vi "PV ModulLine config relay.vi"(8 "error in (no error)":errorcluster, 9 "PV ModulLine config relay - Cluster":T1={"Parameter"=enum." Configuration Relais 1 (045)", "Parameter\nread only<->describe"=FALSE, "Configuration R1 .. R6"=9, "Pressure switch point (hPa)"=1.0000000005} {"Pressure switch point (hPa)" min=5e-10 max=2000.0 step=1.0 format="%_3e"; "Configuration R1 .. R6" items=["0 = rot. speed switch point attained", "1 = no error", "2 = error", "3 = warning", "4 = error and/or warning", "5 = set speed attained", "6 = pump on", "7 = pump accelerates", "8 = pump decelerater", "9 = always 0 (off)", "10 = always 1 (on)", "11 = remote priority active", "12 = heating", "13 = backing pump", "14 = sealing gas", "15 = pumping station", "16 = pump rotates", "17 = pump does not rotate", "18 = TMS temperature engaged  ", "19 = Pressure below pressure switchpoint 1", "20 = Pressure below pressure switchpoint 2", "21 = Pressure below pressure switchpoint 3", "22 = Pressure below pressure switchpoint 4"]}, 10 "Adress of unit":u16=10 max=999 step=1, 11 "VISA session":refnum<visa-resource-name>) -> (0 "error out":errorcluster, 2 "response (data)":string, 3 "dup VISA session":refnum<visa-resource-name>)   [LabVIEW 2021, in "Pfeiffer Vacuum.lvlib"]
doc: "There are 6 parameters available, only one of which can be enabled at a time. \n\n Configuration Relais 1 (045)\n Configuration Relais 2 (046)\n Configuration Relais 3 (047)\n Configuration Relais 4 (048)\n Pressure switch point 1 [mbar] (730)\n Pressure switch point 2 [mbar] (732) \n\n \nNote: Any settings for an parameter that is not selected will be ignored. If a value is out of range, it will be changed to either the upper or the lower limit of the range."
uses:
  <instrlib>/Pfeiffer Vacuum/Pfeiffer Vacuum.lvlib
  <instrlib>/Pfeiffer Vacuum/Public/ModulLine/PV ModulLine config relay - Cluster.ctl
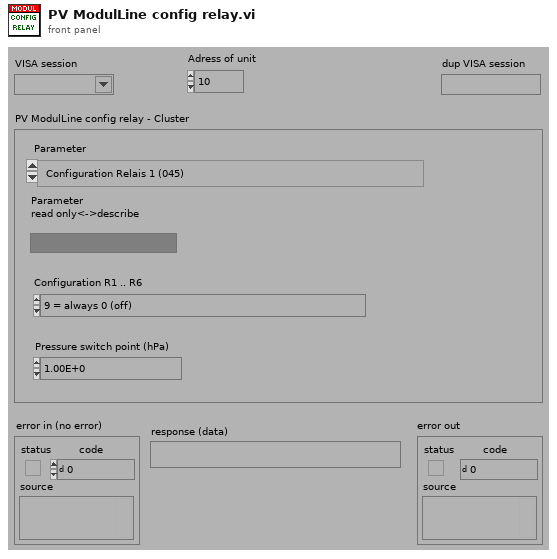
[diagram p1: front panel]
types:
  T1 = typedef "Pfeiffer Vacuum.lvlib/PV ModulLine config relay - Cluster.ctl" = cluster{"Parameter":enum16{" Configuration Relais 1 (045)", " Configuration Relais 2 (046)", " Configuration Relais 3 (047)", " Configuration Relais 4 (048)", " Pressure switch point 1 [mbar] (730)", " Pressure switch point 2 [mbar] (732)"}, "Parameter\nread only<->describe":bool, "Configuration R1 .. R6":u16, "Pressure switch point (hPa)":dbl}
  T2 = enum16{" Configuration Relais 1 (045)", " Configuration Relais 2 (046)", " Configuration Relais 3 (047)", " Configuration Relais 4 (048)", " Pressure switch point 1 [mbar] (730)", " Pressure switch point 2 [mbar] (732)"}
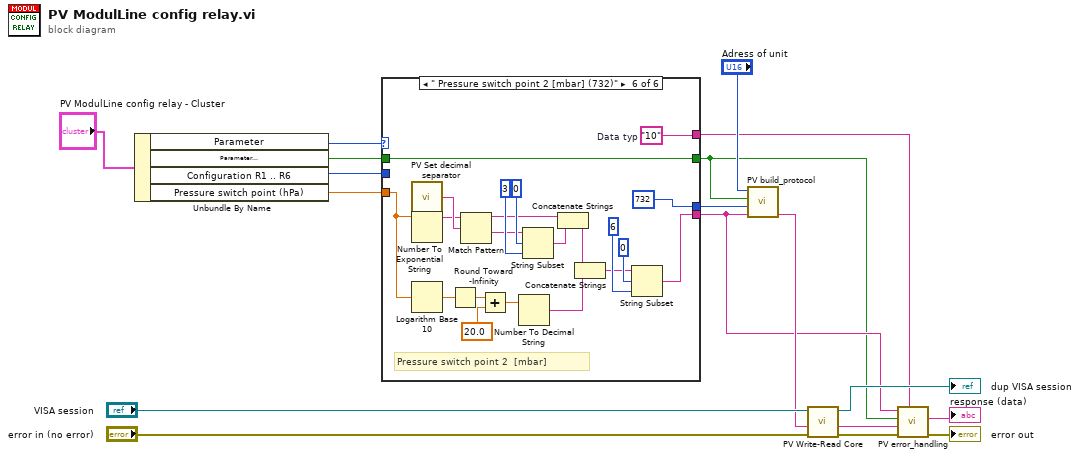
[diagram p0: block diagram]
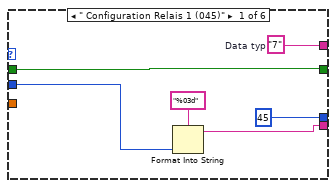
[diagram p2: hidden frame]
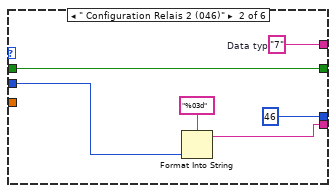
[diagram p3: hidden frame]
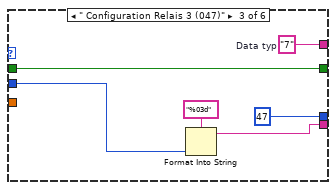
[diagram p4: hidden frame]
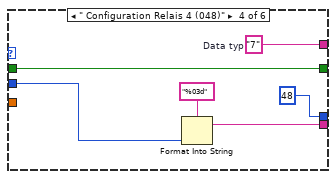
[diagram p5: hidden frame]
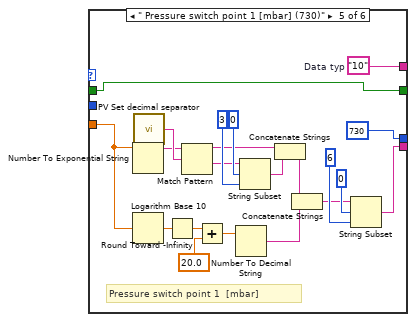
[diagram p6: hidden frame]
diagram:
  n1 = Unbundle By Name("PV ModulLine config relay - Cluster") -> ("Parameter"=w5:T2, "Parameter\nread only<->describe"=w4:bool, "Configuration R1 .. R6"=w3:u16, "Pressure switch point (hPa)"=w1:dbl)
  n2 = case shown="\" Pressure switch point 2 [mbar] (732)\"" w5 {
    tunnel: [u16 45 ("Parameter-number") u16 46 ("Parameter-number") u16 47 ("Parameter-number") u16 48 ("Parameter-number") u16 730 ("Parameter-number") u16 732 ("Parameter-number")] -> w17
    tunnel: [w19 w26 w35 w39 w44 w65] -> w8
    tunnel: [w22 w28 w31 w38 w46 w68] -> w7
    tunnel: [w23 w29 w33 w41 w45 w67] -> w9
    tunnel: w4 -> [w22 w28 w31 w38 w46 w68]
    tunnel: w3 -> [w20 w25 w32 w37 _ _]
    tunnel: w1 -> [_ _ _ _ w47 w64]
    frame " Configuration Relais 1 (045)" {
      w23 = "7"  # Data typ
      n3 = Format Into String(format string="%03d" ("Format-String"), w20) -> (resulting string=w19:string)  [unwired: 2 in, 1 out]
    }
    frame " Configuration Relais 2 (046)" {
      w29 = "7"  # Data typ
      n4 = Format Into String(format string="%03d" ("Format-String"), w25) -> (resulting string=w26:string)  [unwired: 2 in, 1 out]
    }
    frame " Configuration Relais 3 (047)" {
      w33 = "7"  # Data typ
      n5 = Format Into String(format string="%03d" ("Format-String"), w32) -> (resulting string=w35:string)  [unwired: 2 in, 1 out]
    }
    frame " Configuration Relais 4 (048)" {
      w41 = "7"  # Data typ
      n6 = Format Into String(format string="%03d" ("Format-String"), w37) -> (resulting string=w39:string)  [unwired: 2 in, 1 out]
    }
    frame " Pressure switch point 1 [mbar] (730)" {
      w45 = "10"  # Data typ
      # "Pressure switch point 1  [mbar]"
      n7 = Number To Exponential String(number=w47) -> (E-format string=w51:string)  [unwired: 3 in]
      n8 = Logarithm Base 10(1:w47) -> (0:w48:dbl)
      n9 = call <instrlib>:"PV Set decimal separator.vi"() -> ("decimal separator"=w63:string)
      n10 = Round Toward -Infinity(1:w48) -> (0:w49:dbl)
      n11 = Match Pattern(string=w51, regular expression=w63) -> (before substring=w50:string, after substring=w52:string)  [unwired: 1 in, 2 out]
      n12 = Add(x=w49, y=20.0) -> (x+y=w56:dbl)
      n13 = Number To Decimal String(number=w56) -> (decimal integer string=w59:string)  [unwired: 1 in]
      n14 = String Subset(string=w52, offset (0)=0 ("Offset (0)"), length (rest)=3 ("Länge")) -> (substring=w55:string)
      n15 = Concatenate Strings(w50, w55) -> (w58:string)
      n16 = Concatenate Strings(w58, w59) -> (w60:string)
      n17 = String Subset(string=w60, offset (0)=0 ("Offset (0)"), length (rest)=6 ("Länge")) -> (substring=w44:string)
    }
    frame " Pressure switch point 2 [mbar] (732)" {
      w67 = "10"  # Data typ
      # "Pressure switch point 2  [mbar]"
      n18 = call <instrlib>:"PV Set decimal separator.vi"() -> ("decimal separator"=w84:string)
      n19 = Number To Exponential String(number=w64) -> (E-format string=w72:string)  [unwired: 3 in]
      n20 = Logarithm Base 10(1:w64) -> (0:w69:dbl)
      n21 = Round Toward -Infinity(1:w69) -> (0:w70:dbl)
      n22 = Match Pattern(string=w72, regular expression=w84) -> (before substring=w71:string, after substring=w73:string)  [unwired: 1 in, 2 out]
      n23 = Add(x=w70, y=20.0) -> (x+y=w77:dbl)
      n24 = Number To Decimal String(number=w77) -> (decimal integer string=w80:string)  [unwired: 1 in]
      n25 = String Subset(string=w73, offset (0)=0 ("Offset (0)"), length (rest)=3 ("Länge")) -> (substring=w76:string)
      n26 = Concatenate Strings(w71, w76) -> (w79:string)
      n27 = Concatenate Strings(w79, w80) -> (w81:string)
      n28 = String Subset(string=w81, offset (0)=0 ("Offset (0)"), length (rest)=6 ("Länge")) -> (substring=w65:string)
    }
  }
  n29 = call <instrlib>:"PV build_protocol.vi"("Data"=w8, "Parameter-number"=w17, "parameter\nread<->describe"=w7, "Adress"="Adress of unit") -> ("output"=w13:string)  [unwired: 3 in]
  n30 = call <instrlib>:"PV Write-Read Core.vi"("error in"="error in (no error)", "Write data in"=w13, "VISA session"="VISA session") -> ("error out"=w10:errorcluster, "response (data) out"=w11:string, "dup VISA session"=→"dup VISA session":refnum<visa-resource-name>)  [unwired: 2 in]
  n31 = call <instrlib>:"PV error_handling.vi"("Data Typ in"=w9, "error in"=w10, "response (data) in"=w11, "Parameter\nread only<->describe"=w7, "data in"=w8) -> ("error out"=→"error out":errorcluster, "Data out"=→"response (data)":string)  [unwired: 4 in, 1 out]
